vi "Mcp2210 Get Connected Dev Count net4.vi"(8 "error in (no error)":errorcluster, 10 "pid":u16 format="%x", 11 "vid":u16 format="%x") -> (0 "error out":errorcluster, 3 "Number of Devices":i32)   [LabVIEW 2015, in "mcp2210.lvlib"]
doc: "provides the number of connected devices with the given VID:PID.\nReturns negative number in case of error.\nParameters:\nInputs:\n- unsigned short vid - MCP2210 device VendorID (Microchip default = 0x4D8)\n- unsigned short pid - MCP2210 device ProductID (Microchip default = 0xDE)\nOutputs:\n- none\nReturns:\n- the number of connected devices with the given VID:PID or\n- negative error code: M_E_ERR_UNKOWN_ERROR, M_E_ERR_MALLOC\n\nMCP2210_DLL_UM_API int __stdcall Mcp2210_GetConnectedDevCount(unsigned short vid, unsigned short pid);"
uses:
  <userlib>/mcp2210/mcp2210.lvlib
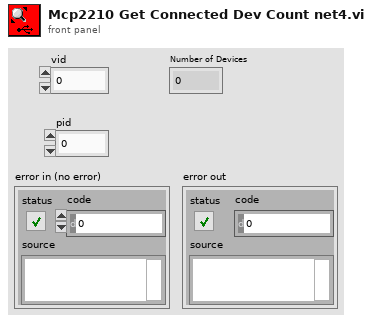
[diagram p1: front panel]
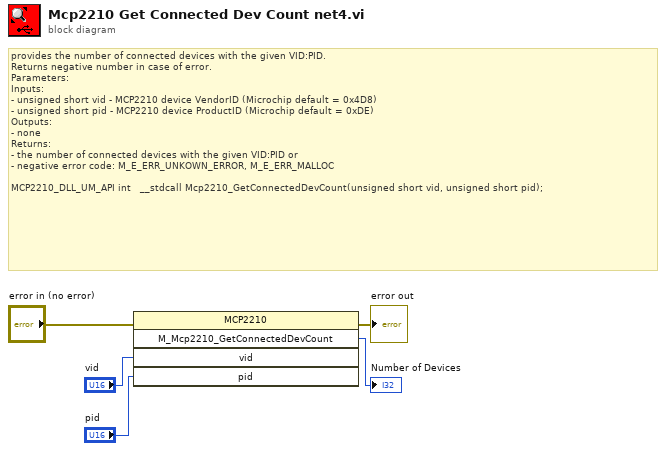
[diagram p0: block diagram]
diagram:
  # "provides the number of connected devices with the given VID:PID.\nReturns negative number in case of error.\nParameters:\nInputs:\n- unsigned short vid - MCP2210 device VendorID (Microchip default = 0x4D8)\n- unsigned short pid - MCP2210 device ProductID (Microchip default = 0xDE)\nOutputs:\n- none\nReturns:\n- the number of connected devices with the given VID:PID or\n- negative error code: M_E_ERR_UNKOWN_ERROR, M_E_ERR_MALLOC\n\nMCP2210_DLL_UM_API int   __stdcall Mcp2210_GetConnectedDevCount(unsigned short vid, unsigned short pid);"
  n1 = invoke class="MCP2210" method="M_Mcp2210_GetConnectedDevCount"(error in="error in (no error)", "vid"="vid", "pid"="pid") -> (error out=→"error out":errorcluster, "M_Mcp2210_GetConnectedDevCount"=→"Number of Devices":i32)  [unwired: 2 in, 3 out]
